vi "RSZVB Define PAE Measurement.vi"(6 "Constant c (0.0 W/V)":dbl format="%^.3e", 7 "Constant k (0.0 W/V^2)":dbl format="%^.3e", 8 "error in (no error)":errorcluster {"code" format="%.0x"}, 9 "Test Model (0: c * U (DC Meas +/-10 V))":i32(ring) items=["c * U (DC Meas +/-10 V)", "c * U (DC Meas +/-1 V)", "k * U (DC Meas +/-10 V) * U (DC Meas +/-1 V)", "c * U (DC Meas +/-1 V) - k * U (DC Meas +/-1 V)^2"], 10 "Channel (Trace) (1)":i32=1, 11 "VISA session":refnum<visa-resource-name>) -> (0 "error out":errorcluster {"code" format="%.0x"}, 3 "dup VISA session":refnum<visa-resource-name>)   [LabVIEW 2011]
doc: "This VI select the test model and the parameters for measuring the DC power PDC supplied to the DUT.\n\nThe power PDC supplied to the DUT can be measured using either one of the DC inputs DC MEAS +/-10V (for large voltages), DC MEAS +/-1V (for small voltages) or both inputs. Define DC Power Measurement in the PAE measurement suggests different models involving different test setups and approximations.\n\nRemote-control command(s):\n[SENSe<Ch/Tr>:]PAE:EXPRession C10 | C1 | K101 | CK11\n[SENSe<Ch/Tr>:]PAE:C <numeric_value>\n[SENSe<Ch/Tr>:]PAE:K <numeric_value>"
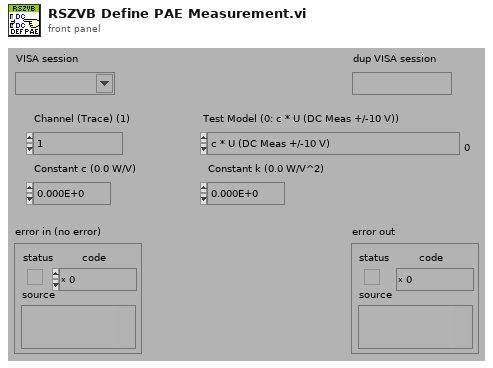
[diagram p1: front panel]
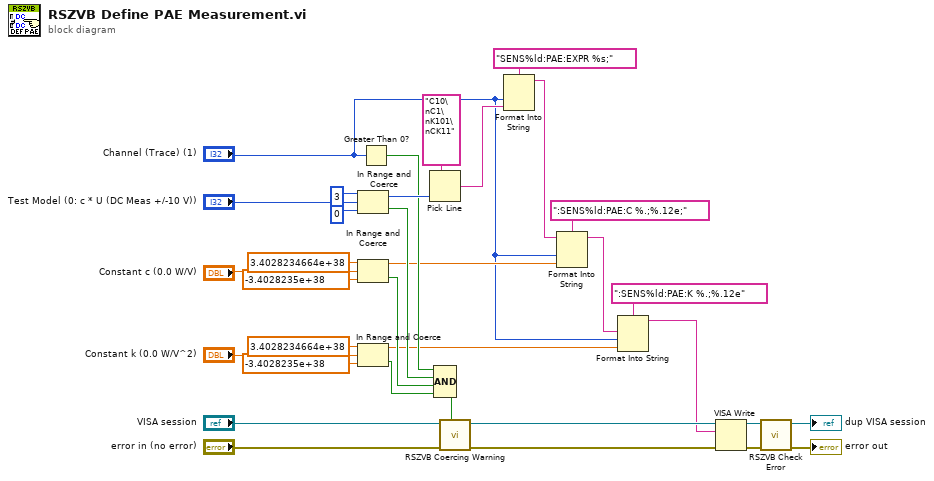
[diagram p0: block diagram]
diagram:
  n1 = In Range and Coerce(upper limit=3, x="Test Model (0: c * U (DC Meas +/-10 V))", lower limit=0) -> (coerced(x)=w14:i32, In Range?=w12:bool)
  n2 = In Range and Coerce(upper limit=3.4028234664e+38, x="Constant c (0.0 W/V)", lower limit=-3.4028235e+38) -> (coerced(x)=w2:dbl, In Range?=w11:bool)
  n3 = In Range and Coerce(upper limit=3.4028234664e+38, x="Constant k (0.0 W/V^2)", lower limit=-3.4028235e+38) -> (coerced(x)=w3:dbl, In Range?=w10:bool)
  n4 = Greater Than 0?(x="Channel (Trace) (1)") -> (x > 0?=w13:bool)
  n5 = Pick Line(multi-line string="C10\nC1\nK101\nCK11", line index=w14) -> (output string=w15:string)  [unwired: 1 in]
  n6 = Compound Arithmetic op=AND(w13, w12, w11, w10) -> (w9:bool)
  n7 = call "RSZVB Coercing Warning.vi"("In Range?"=w9, "error in (no error)"="error in (no error)", "VISA session"="VISA session") -> ("error out"=w33:errorcluster, "dup VISA session"=w34:refnum<visa-resource-name>)  [unwired: 7 in]
  n8 = Format Into String(format string="SENS%ld:PAE:EXPR %s;", "Channel (Trace) (1)", w15) -> (resulting string=w5:string)  [unwired: 2 in, 1 out]
  n9 = Format Into String(format string=":SENS%ld:PAE:C %.;%.12e;", initial string=w5, "Channel (Trace) (1)", w2) -> (resulting string=w4:string)  [unwired: 1 in, 1 out]
  n10 = Format Into String(format string=":SENS%ld:PAE:K %.;%.12e", initial string=w4, "Channel (Trace) (1)", w3) -> (resulting string=w6:string)  [unwired: 1 in, 1 out]
  n11 = VISA Write(VISA resource name=w34, write buffer=w6, error in (no error)=w33) -> (VISA resource name out=w7:refnum<visa-resource-name>, error out=w8:errorcluster)  [unwired: 1 out]
  n12 = call "RSZVB Check Error.vi"("error in (no error)"=w8, "VISA session"=w7) -> ("error out"=→"error out":errorcluster, "dup VISA session"=→"dup VISA session":refnum<visa-resource-name>)  [unwired: 8 in]
